vi "dequeue.vi"(8 "error in (no error)":errorcluster, 11 "EventDaemon in":refnum<class "ErrorHandler.lvclass">) -> (0 "error out":errorcluster, 2 "state":T1, 3 "EventDaemon out":refnum<class "ErrorHandler.lvclass">, 5 "timeout":i32)   [LabVIEW 2024, in "ErrorHandler.lvclass"]
doc: "Dequeues private states for daemon."
uses:
  ErrorHandler.lvclass
  ErrorHandler.lvclass/ErrorHandler.ctl
  states--enum.ctl
panel:
  out "data":errorcluster
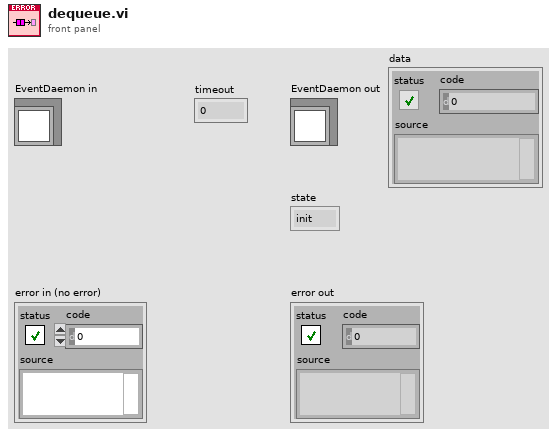
[diagram p1: front panel]
types:
  T1 = typedef "ErrorHandler.lvclass/states--enum.ctl" = enum16{"init", "default", "display error", "error handler", "exit"}
  T2 = typedef "ErrorHandler.lvclass/msg--cluster.ctl" = cluster{"cmd":T1, "error":errorcluster}
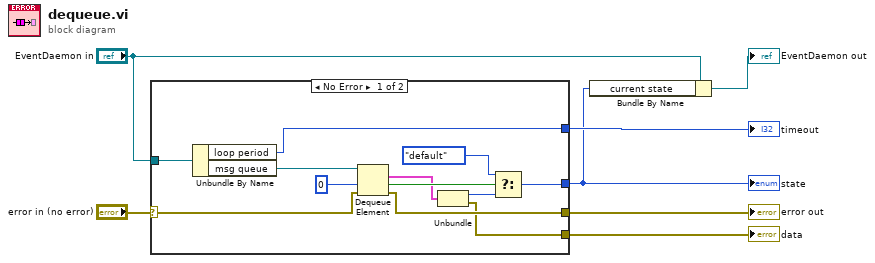
[diagram p0: block diagram]
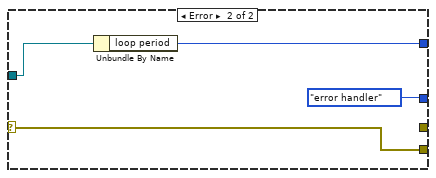
[diagram p2: hidden frame]
diagram:
  n1 = case shown="No Error" "error in (no error)" {
    selector: "error in (no error)" -> [w12 w20]
    tunnel: "EventDaemon in" -> [w19 w22]
    tunnel: [w16 _] -> w7
    tunnel: [w13 states--enum."error handler" ("states")] -> w2
    tunnel: [w11 w21] -> w5
    tunnel: [w8 w20] -> w1
    frame No Error {
      n2 = Unbundle By Name(w19) -> ("loop period"=w11:i32, "msg queue"=w18:refnum<queue>)
      n3 = Dequeue Element(queue=w18, timeout in ms (-1)=0, error in (no error)=w12) -> (element=w10:T2, timed out?=w15:bool, error out=w16:errorcluster)  [unwired: 1 out]
      n4 = Unbundle(w10) -> ("cmd"=w9:T1, "error"=w8:errorcluster)
      n5 = Select(t=states--enum."default", s=w15, f=w9) -> (s? t:f=w13:T1)
    }
    frame Error {
      n6 = Unbundle By Name(w22) -> ("loop period"=w21:i32)
    }
  }
  "error out" <- w7
  "state" <- w2
  "timeout" <- w5
  "data" <- w1
  n7 = Bundle By Name(cluster="EventDaemon in", "current state"=w2) -> (→"EventDaemon out":refnum<class "ErrorHandler.lvclass">)
